vi "Complete Pattern Script.vi"(8 "error in (no error)":errorcluster, 9 "Pattern Contents":string, 10 "Pattern Name":string, 11 "BML_DigiPattern_Generator.lvclass":refnum<class "BML_DigiPattern_Generator.lvclass">) -> (0 "error out":errorcluster, 2 "All Pattern Script out":string, 3 "BML_DigiPattern_Generator.lvclass out":refnum<class "BML_DigiPattern_Generator.lvclass">)   [LabVIEW 2016, in "BML_DigiPattern_Generator.lvclass"]
uses:
  BML_DigiPattern_Generator.lvclass
  BML_Frame_Root/BML_Frame_Root.lvclass
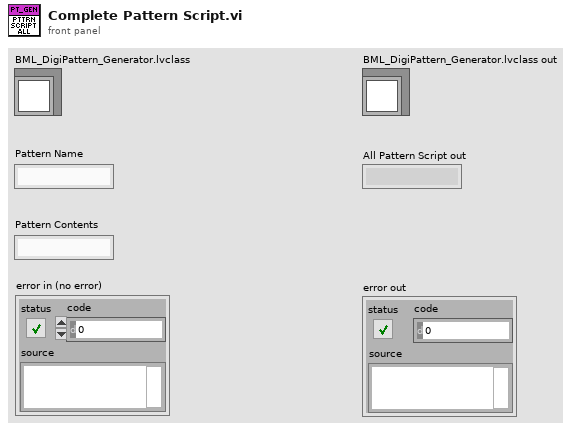
[diagram p1: front panel]
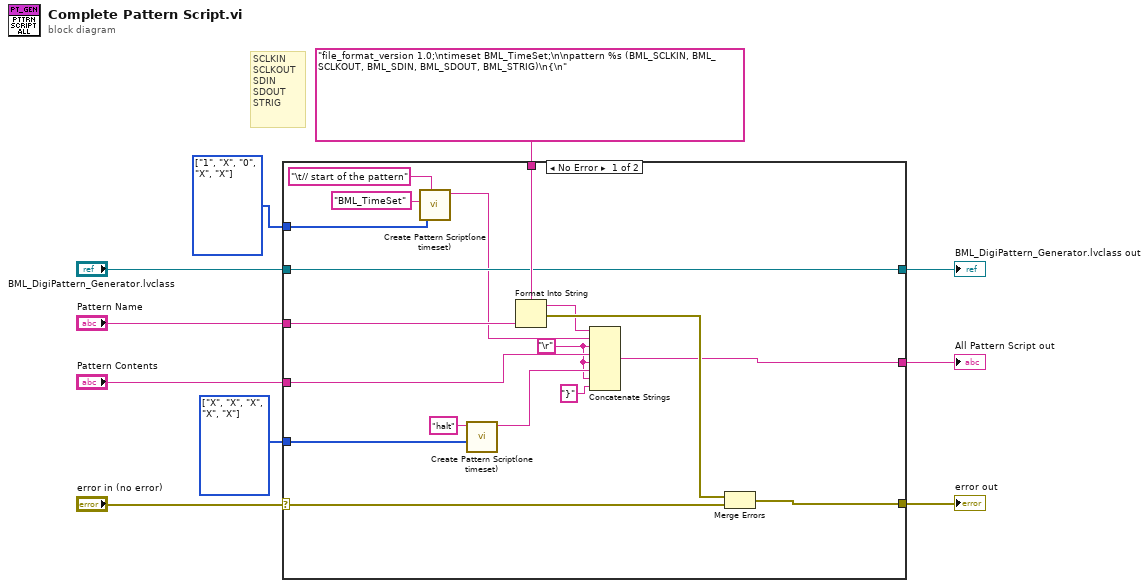
[diagram p0: block diagram]
diagram:
  w1 = enum16{"0", "1", "L", "H", "X", "V", "D", "M"}[] [enum."X", enum."X", enum."X", enum."X", enum."X"] items=["0", "1", "L", "H", "X", "V", "D", "M"] ("PinState")
  w2 = enum16{"0", "1", "L", "H", "X", "V", "D", "M"}[] [enum."1", enum."X", enum."0", enum."X", enum."X"] items=["0", "1", "L", "H", "X", "V", "D", "M"] ("PinState")
  # "SCLKIN\nSCLKOUT\nSDIN\nSDOUT\nSTRIG"
  n1 = case shown="No Error" "error in (no error)" {
    selector: "error in (no error)" -> [w24 w30]
    tunnel: "BML_DigiPattern_Generator.lvclass" -> [w22 w29]
    tunnel: [w23 w30] -> w8
    tunnel: [w22 w29] -> w7
    tunnel: "Pattern Name" -> [w27 _]
    tunnel: "Pattern Contents" -> [w26 _]
    tunnel: "file_format_version 1.0;\ntimeset BML_TimeSet;\n\npattern %s (BML_SCLKIN, BML_SCLKOUT, BML_SDIN, BML_SDOUT, BML_STRIG)\n{\n" -> [w28 _]
    tunnel: [w21 _] -> w3
    tunnel: w2 -> [w19 _]
    tunnel: w1 -> [w14 _]
    frame No Error {
      w12 = "\r"
      n2 = call "Create Pattern Script(one timeset).vi"("Notes"="\t// start of the pattern", "PinState"=w19, "timeset name"="BML_TimeSet") -> ("string out"=w16:string)  [unwired: 8 in]
      n3 = call "Create Pattern Script(one timeset).vi"("PinState"=w14, "opcode"="halt") -> ("string out"=w15:string)  [unwired: 9 in]
      n4 = Format Into String(format string=w28, w27) -> (resulting string=w17:string, error out=w25:errorcluster)  [unwired: 2 in]
      n5 = Concatenate Strings(w17, w16, w12, w26, w12, w15, w12, "}") -> (w21:string)
      n6 = Merge Errors(w25, w24) -> (w23:errorcluster)
    }
    frame Error {
    }
  }
  "error out" <- w8
  "BML_DigiPattern_Generator.lvclass out" <- w7
  "All Pattern Script out" <- w3
